vi "Wait for answer 0 or 1 without polling.vi"(0 "System no.":i32=1 min=1 max=4 step=1, 5 "error in":errorcluster, 10 "Start time":dbl format="%.2f", 11 "Timeout (s)":dbl=60.0 format="%.2f", 12 "Stop refnum":refnum<vi>) -> (14 "Scan successful?":bool, 15 "Stopped":bool, 19 "error out":errorcluster)   [LabVIEW 2026]
doc: "This VI waits until answer 0 or 1 comes or timeout is reached without single character polling. VI also stops if Stop refnum or Local stop is TRUE. When using as a sub-VI, use Stop refnum to stop VI from caller."
uses:
  Communication/Global1.vi
panel:
  in  "Local stop":bool
  # "This vi waits until answer 0 or 1 comes, Stop refnum or Local stop is \nTRUE, or timeout is reached."
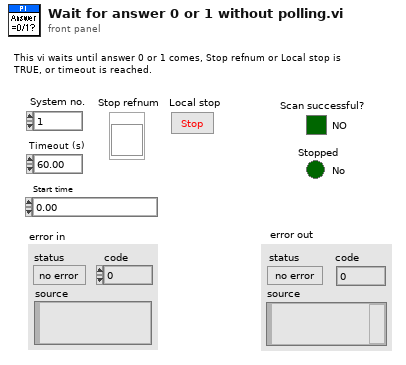
[diagram p1: front panel]
types:
  T1 = typedef "Semaphore RefNum" = refnum<k1>
  T2 = typedef "Available interfaces.ctl" = u16
  T3 = cluster{"RS232 Portnumber":i32, "Timeout":i32, "RS232 Baud rate":u32, "Interface":T2, "GPIB Bus":i32, "GPIB Address":i32, "GPIB Mode":i32}[]
  T4 = cluster{"RS232 Portnumber":i32, "Timeout":i32, "RS232 Baud rate":u32, "Interface":T2, "GPIB Bus":i32, "GPIB Address":i32, "GPIB Mode":i32}
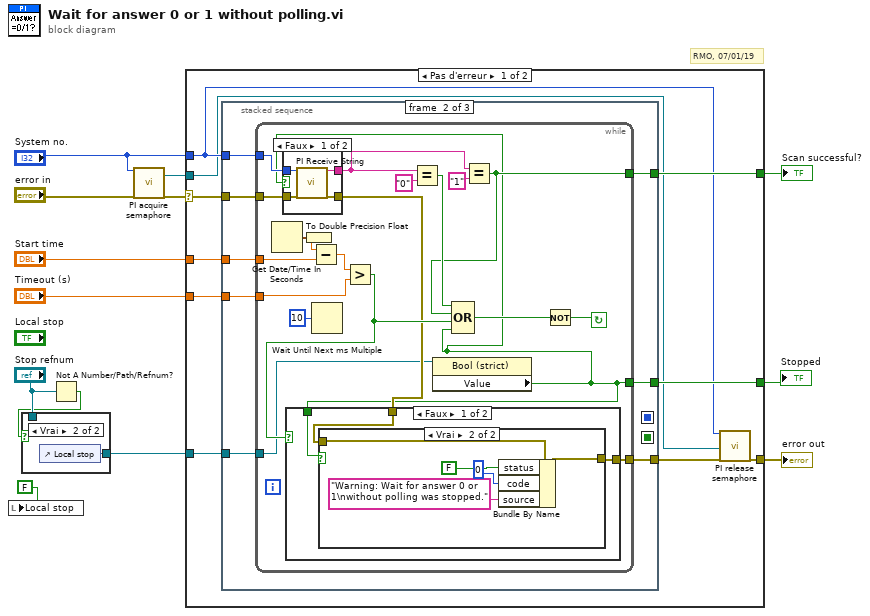
[diagram p0: block diagram]
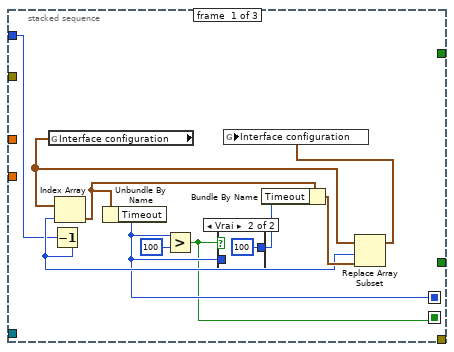
[diagram p3: hidden frame]
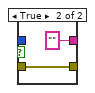
[diagram p5: hidden frame]
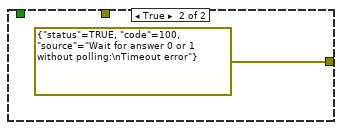
[diagram p7: hidden frame]
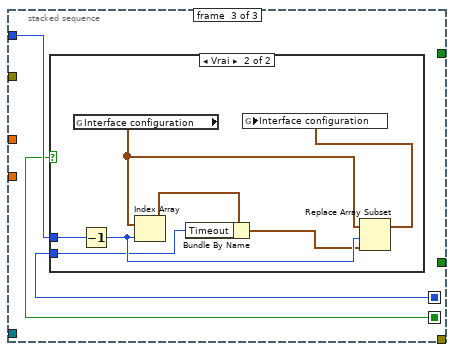
[diagram p8: hidden frame]
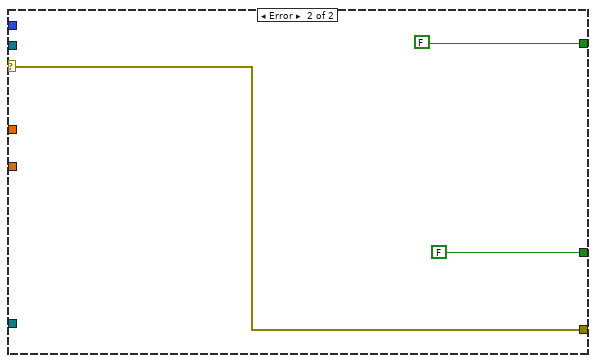
[diagram p10: hidden frame]
diagram:
  # "RMO, 07/01/19"
  n1 = local write "Local stop"(FALSE ("Local stop")) -> ()
  n2 = Not A Number/Path/Refnum?(number/path/refnum="Stop refnum") -> (NaN/Path/Refnum?=w8:bool)
  n3 = case shown="Vrai" w8 {
    tunnel: [w14 w15] -> w7
    tunnel: "Stop refnum" -> [w14 _]
    frame False {
    }
    frame True {
      n4 = control-ref of="Local stop"() -> (w15:refnum<vi>)
    }
  }
  n5 = call "PI acquire semaphore.vi"("System no."="System no.", "error in"="error in") -> ("semaphore out"=w1:T1, "error out"=w2:errorcluster)  [unwired: 16 out]
  n6 = case shown="Pas d'erreur" w2 {
    selector: w2 -> [w20 w92]
    tunnel: "Timeout (s)" -> [w25 _]
    tunnel: "Start time" -> [w24 _]
    tunnel: "System no." -> [w17 _]
    tunnel: [w23 FALSE] -> w11
    tunnel: [w18 w92] -> w10
    tunnel: w7 -> [w22 _]
    tunnel: [w21 FALSE ("Value")] -> w5
    tunnel: w1 -> [w16 _]
    frame No Error {
      n7 = stacked-sequence {
        seq-local: [w27 _ _] -> [_ _ w84]
        seq-local: [w26 _ _] -> [_ _ w82]
        tunnel: w25 -> [_ w45 _]
        tunnel: w24 -> [_ w44 _]
        tunnel: w17 -> [w28 w43 w83]
        tunnel: [_ w42 _] -> w23
        tunnel: [_ w41 _] -> w19
        tunnel: w20 -> [_ w40 _]
        tunnel: w22 -> [_ w39 _]
        tunnel: [_ w38 _] -> w21
        frame #0 {
          n8 = global read "Global1.vi" "Interface configuration"() -> (w32:T3)
          n9 = Decrement(x=w28) -> (x-1=w34:i32)
          n10 = Index Array(array=w32, index=w34) -> (element=w31:T4)
          n11 = Unbundle By Name(w31) -> ("Timeout"=w27:i32)
          n12 = Greater?(x=w27, y=u32 100) -> (0:w26:bool)
          n13 = case shown="Vrai" w26 {
            tunnel: [w36 100] -> w30
            tunnel: w27 -> [w36 _]
            frame False {
            }
            frame True {
            }
          }
          n14 = Bundle By Name(cluster=w31, "Timeout"=w30) -> (w35:T4)
          n15 = Replace Array Subset(array=w32, new element=w35, index=w34) -> (w33:T3)
          n16 = global write "Global1.vi" "Interface configuration"(w33) -> ()
        }
        frame #1 {
          n17 = while {
            tunnel: [w46] -> w38
            tunnel: w39 -> [w50]
            tunnel: [w51] -> w41
            tunnel: w43 -> [w54]
            tunnel: w40 -> [w55]
            tunnel: [w57] -> w42
            tunnel: w45 -> [w60]
            tunnel: w44 -> [w62]
            stop <- w64 continue-if-true
            n18 = Get Date/Time In Seconds() -> (seconds since 1Jan1904=w49:timestamp)
            n19 = To Double Precision Float(number=w49) -> (double precision float=w63:dbl)
            n20 = Subtract(x=w63, y=w62) -> (x-y=w61:dbl)
            n21 = Wait Until Next ms Multiple(millisecond multiple=u32 10) -> ()  [unwired: 1 out]
            n22 = Greater?(x=w61, y=w60) -> (0:w53:bool)
            n23 = property class="Bool (strict)"(reference=w50) -> ("Value"=w46:bool)  [unwired: 1 in, 2 out]
            n24 = case shown="Faux" w46 {
              tunnel: [w69 "" ("String read")] -> w58
              tunnel: w55 -> [w68 w70]
              tunnel: w54 -> [w67 _]
              tunnel: [w66 w70] -> w52
              frame False {
                n25 = call "PI Receive String.vi"("System no."=w67, "error in"=w68) -> ("String read"=w69:string, "error out"=w66:errorcluster)  [unwired: 1 in, 15 out]
              }
              frame True {
              }
            }
            n26 = case shown="Faux" w53 {
              tunnel: [w74 errorcluster {"status"=TRUE, "code"=100, "source"="Wait for answer 0 or 1 without polling:\nTimeout error"} ("error out")] -> w51
              tunnel: w52 -> [w73 _]
              tunnel: w46 -> [w72 _]
              frame False {
                n27 = case shown="Vrai" w72 {
                  tunnel: [w75 w79] -> w74
                  tunnel: w73 -> [w75 w80]
                  frame False {
                  }
                  frame True {
                    n28 = Bundle By Name(cluster=w80, "status"=FALSE, "code"=0, "source"="Warning: Wait for answer 0 or 1\nwithout polling was stopped.") -> (w79:errorcluster)
                  }
                }
              }
              frame True {
              }
            }
            n29 = Equal?(x=w58, y="0") -> (x = y?=w59:bool)
            n30 = Equal?(x=w58, y="1") -> (x = y?=w57:bool)
            n31 = Compound Arithmetic op=OR(w59, w57, w53, w46) -> (w65:bool)
            n32 = Not(x=w65) -> (.not. x?=w64:bool)
          }
        }
        frame #2 {
          n33 = case shown="Vrai" w82 {
            tunnel: w83 -> [_ w90]
            tunnel: w84 -> [_ w85]
            frame False {
            }
            frame True {
              n34 = global read "Global1.vi" "Interface configuration"() -> (w89:T3)
              n35 = Decrement(x=w90) -> (x-1=w87:i32)
              n36 = Index Array(array=w89, index=w87) -> (element=w91:T4)
              n37 = Bundle By Name(cluster=w91, "Timeout"=w85) -> (w86:T4)
              n38 = Replace Array Subset(array=w89, new element=w86, index=w87) -> (w88:T3)
              n39 = global write "Global1.vi" "Interface configuration"(w88) -> ()
            }
          }
        }
      }
      n40 = call "PI release semaphore.vi"("System no."=w17, "semaphore"=w16, "error in"=w19) -> ("error out"=w18:errorcluster)  [unwired: 1 in, 15 out]
    }
    frame Error {
    }
  }
  "Scan successful?" <- w11
  "error out" <- w10
  "Stopped" <- w5
